vi "ACTION.vi"(8 "error in (no error)":errorcluster, 9 "STEP State":T1, 10 "CORE":refnum<queue>, 11 "Relev in":refnum<class "Relev.lvclass">) -> (0 "error out":errorcluster, 3 "Relev out":refnum<class "Relev.lvclass">)   [LabVIEW 2014, in "SeqLoop.lvlib" / "STEP Classes.lvlib" / "Relev.lvclass"]
uses:
  Relev.lvclass
  TypeDefs/STEP State.ctl
  APIs/Message Queue/Message Cluster.ctl
  Relev.lvclass/Relev.ctl
  APIs/Message Queue/Enqueue Message (Array).vi
  APIs/Message Queue/Enqueue Message (Single).vi
  APIs/Message Queue/WINFAS 2 Message Queue.lvlib
  SeqLoop.lvlib
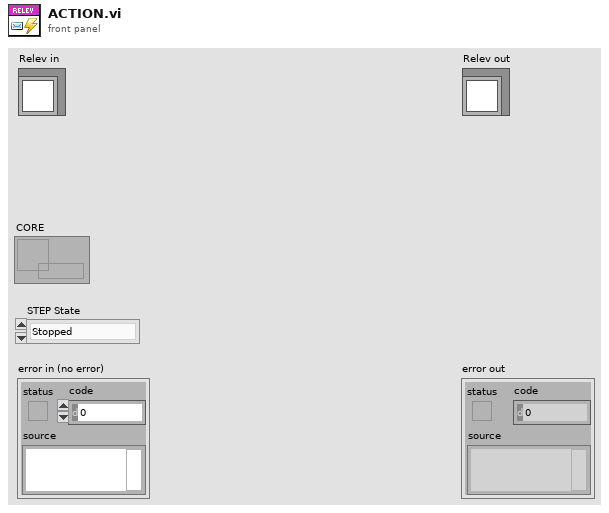
[diagram p1: front panel]
types:
  T1 = typedef "SeqLoop.lvlib/STEP State.ctl" = enum16{"Stopped", "First Call", "Idle...", "Advance OK", "Alarm", "Output Security", "Error"}
  T2 = cluster{"HWSync 1":bool, "HWSync 2":bool, "HWSync 3":bool, "HWSync 4":bool, "HWSync 5":bool}
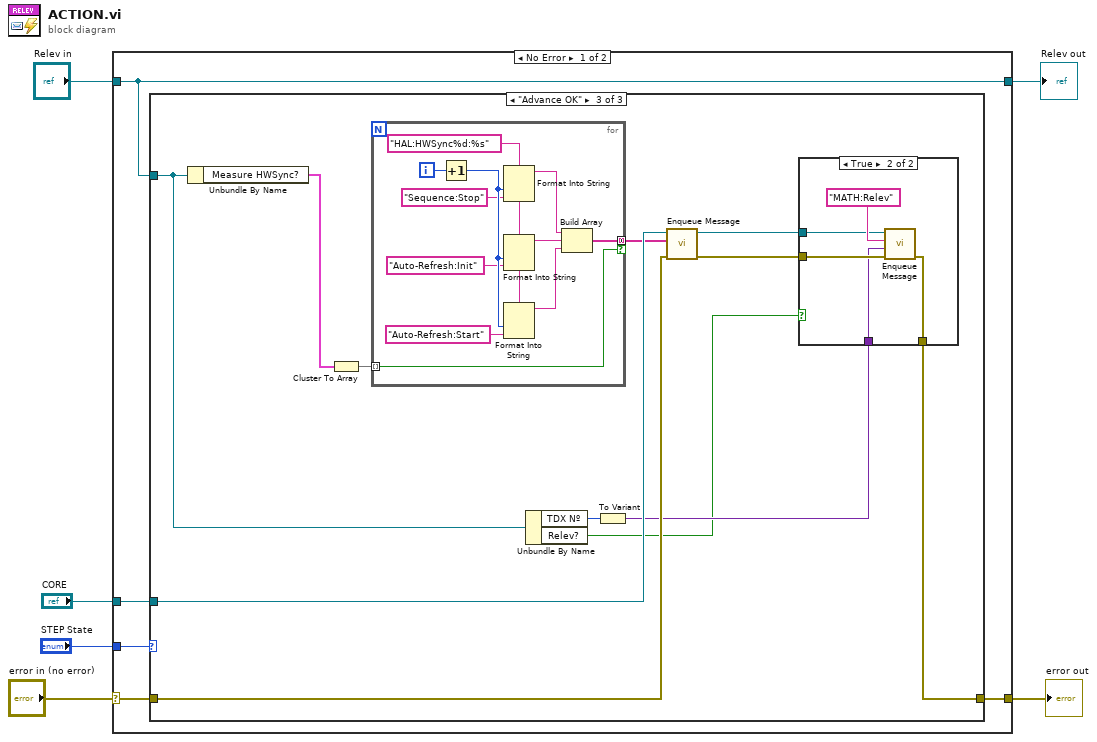
[diagram p0: block diagram]
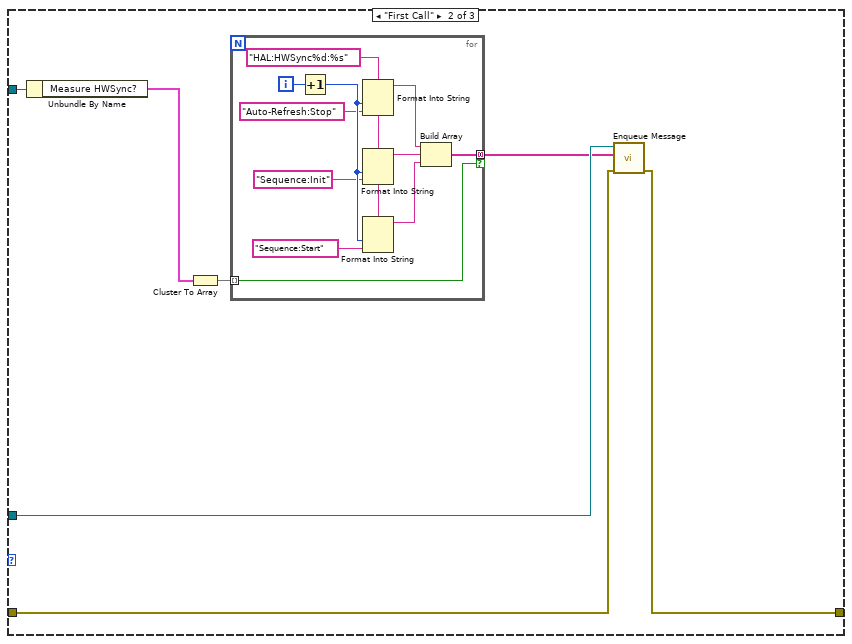
[diagram p3: hidden frame]
diagram:
  n1 = case shown="No Error" "error in (no error)" {
    selector: "error in (no error)" -> [w8 w61]
    tunnel: [w7 w61] -> w1
    tunnel: [w9 w60] -> w5
    tunnel: "Relev in" -> [w9 w60]
    tunnel: "CORE" -> [w10 _]
    tunnel: "STEP State" -> [w11 _]
    frame No Error {
      n2 = case shown="\"Advance OK\"" w11 {
        tunnel: w10 -> [_ w16 w40]
        tunnel: w9 -> [_ w18 w32]
        tunnel: w8 -> [w12 w15 w39]
        tunnel: [w12 w14 w36] -> w7
        frame Default {
        }
        frame "First Call" {
          n3 = Unbundle By Name(w18) -> ("Measure HWSync?"=w17:T2)
          n4 = Cluster To Array(cluster=w17) -> (array=w19:bool[])
          n5 = for {
            tunnel: w19 -> [w20] mode=indexing
            tunnel: [w21] -> w13 mode=concatenating if=w20
            i -> [w30]
            w29 = "HAL:HWSync%d:%s" ("format string")
            n6 = Increment(x=w30) -> (x+1=w28:i32)
            n7 = Format Into String(format string=w29, w28, "Auto-Refresh:Stop" ("format string")) -> (resulting string=w24:string)  [unwired: 2 in, 1 out]
            n8 = Format Into String(format string=w29, w28, "Sequence:Init" ("format string")) -> (resulting string=w23:string)  [unwired: 2 in, 1 out]
            n9 = Format Into String(format string=w29, w28, "Sequence:Start" ("format string")) -> (resulting string=w22:string)  [unwired: 2 in, 1 out]
            n10 = Build Array(w24, w23, w22) -> (w21:string[])
          }
          n11 = call-poly "Enqueue Message.vi"("error in (no error)"=w15, "Message Array"=w13, "Message Queue"=w16) -> ("error out"=w14:errorcluster)  [unwired: 7 in, 1 out]
        }
        frame "Advance OK" {
          n12 = Unbundle By Name(w32) -> ("Measure HWSync?"=w41:T2)
          n13 = Cluster To Array(cluster=w41) -> (array=w42:bool[])
          n14 = for {
            tunnel: w42 -> [w49] mode=indexing
            tunnel: [w50] -> w38 mode=concatenating if=w49
            i -> [w59]
            w58 = "HAL:HWSync%d:%s" ("format string")
            n15 = Increment(x=w59) -> (x+1=w57:i32)
            n16 = Format Into String(format string=w58, w57, "Sequence:Stop" ("format string")) -> (resulting string=w53:string)  [unwired: 2 in, 1 out]
            n17 = Format Into String(format string=w58, w57, "Auto-Refresh:Init" ("format string")) -> (resulting string=w52:string)  [unwired: 2 in, 1 out]
            n18 = Format Into String(format string=w58, w57, "Auto-Refresh:Start" ("format string")) -> (resulting string=w51:string)  [unwired: 2 in, 1 out]
            n19 = Build Array(w53, w52, w51) -> (w50:string[])
          }
          n20 = Unbundle By Name(w32) -> ("TDX Nº"=w34:i32, "Relev?"=w31:bool)
          n21 = To Variant(anything=w34) -> (Variant=w33:variant)
          n22 = call-poly "Enqueue Message.vi"("error in (no error)"=w39, "Message Array"=w38, "Message Queue"=w40) -> ("error out"=w37:errorcluster, "dup Message Queue"=w35:refnum<queue>)  [unwired: 7 in]
          n23 = case shown="True" w31 {
            tunnel: w37 -> [w43 w48]
            tunnel: [w43 w47] -> w36
            tunnel: w35 -> [_ w45]
            tunnel: w33 -> [_ w44]
            frame False {
            }
            frame True {
              n24 = call-poly "Enqueue Message.vi"("error in (no error)"=w48, "Message Data"=w44, "Message"="MATH:Relev" ("format string"), "Message Queue"=w45) -> ("error out"=w47:errorcluster)  [unwired: 6 in, 1 out]
            }
          }
        }
      }
    }
    frame Error {
    }
  }
  "error out" <- w1
  "Relev out" <- w5
